vi "c Spark Register Id.vi"(8 "error in (no error)":errorcluster, 10 "deviceId":i32, 11 "busID":i32) -> (0 "error out":errorcluster, 3 "function return":T1)   [LabVIEW 2023, in "REVLibDriver.lvlib"]
doc: "c_REVLib_ErrorCode c_Spark_RegisterId(int deviceId);"
uses:
  <vilib>/REVLibDriver5/REVLibDriver.lvlib
  lib/libREVLibDriver.so
  <vilib>/REVLibDriver5/subvi/RevLibError.ctl
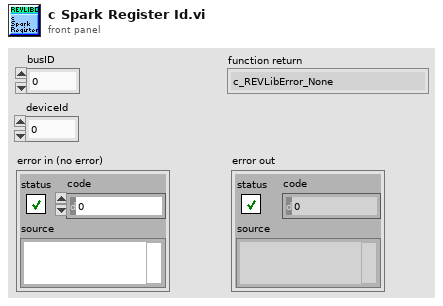
[diagram p1: front panel]
types:
  T1 = typedef "REVLibDriver.lvlib/RevLibError.ctl" = enum16{"c_REVLibError_None", "c_REVLibError_General", "c_REVLibError_CANTimeout", "c_REVLibError_NotImplemented", "c_REVLibError_HAL", "c_REVLibError_CantFindFirmware", "c_REVLibError_FirmwareTooOld", "c_REVLibError_FirmwareTooNew", "c_REVLibError_ParamInvalidID", "c_REVLibError_ParamMismatchType", "c_REVLibError_ParamAccessMode", "c_REVLibError_ParamInvalid", "c_REVLibError_ParamNotImplementedDeprecated", "c_REVLibError_FollowConfigMismatch", "c_REVLibError_Invalid", "c_REVLibError_SetpointOutOfRange", "c_REVLibError_Unknown", "c_REVLibError_CANDisconnected", "c_REVLibError_DuplicateCANId", "c_REVLibError_InvalidCANId", "c_REVLibError_SparkMaxDataPortAlreadyConfiguredDifferently", "c_REVLibError_SparkFlexBrushedWithoutDock", "c_REVLibError_NumCodes"}
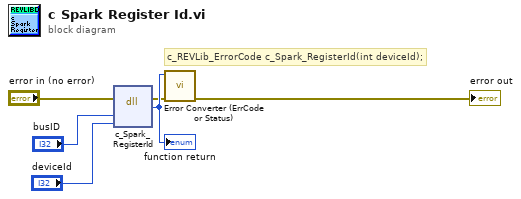
[diagram p0: block diagram]
diagram:
  # "c_REVLib_ErrorCode c_Spark_RegisterId(int deviceId);"
  n1 = dll-call lib="home/systemcore/natinst/lib/libREVLibDriver.so" fn="c_Spark_RegisterId"(error in="error in (no error)", "busId"="busID", "deviceID"="deviceId") -> (error out=w3:errorcluster, "return type"=w6:u32)  [unwired: 4 in, 1 out]
  "function return" <- w6
  n2 = call <vilib>:"Error Converter (ErrCode or Status).vi"("error in (no error)"=w3, "error code"=w6) -> ("error out"=→"error out":errorcluster)  [unwired: 9 in]
